vi "niDTS WLAN INSTR TX Configure ModAcc.vi"(8 "error in (no error)":errorcluster, 11 "niDTS WLAN INSTR TX in":refnum<class "niDTS WLAN INSTR TX.lvclass">) -> (0 "error out":errorcluster, 3 "niDTS WLAN INSTR TX out":refnum<class "niDTS WLAN INSTR TX.lvclass">)   [LabVIEW 2015, in "niDTS WLAN.lvlib" / "niDTS WLAN INSTR TX.lvclass"]
doc: "Sets:\n\n* ModulationEnabled\n* HeaderDetectionEnabled\n* AmplitudeTracking\n* ChannelTracking\n* TimeTracking\n* NumberOfAverages(mod)\n* PayloadLength\n\nNotes: This section is missing Number of Symbols to Analyze and L-SIG length."
uses:
  niDTS WLAN INSTR TX.lvclass
  niDTS WLAN INSTR TX.lvclass/niDTS WLAN INSTR TX.ctl
  RiviInstDriver/niRfsaWlan/Objects/niRfsaWlan.lvclass
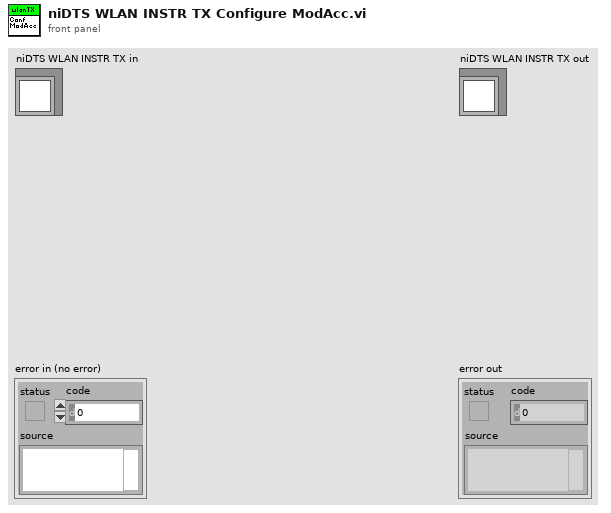
[diagram p1: front panel]
types:
  T1 = typedef "niDTS WLAN.lvlib/niDTS WLAN INC Standard.ctl" = enum16{"802.11 b DSSS", "802.11 a/g OFDM", "802.11 n HT", "802.11 ac VHT"}
  T2 = typedef "niRfsaWlan.lvclass/niRfsaWlan INC Handle.ctl" = refnum<data-value>
  T3 = typedef "niDTS WLAN.lvlib/niDTS WLAN INC DSSS ModAcc Measurement Parameters.ctl" = cluster{"DC Offset Compensation":bool, "Equalization":bool, "Phase Tracking":bool, "Chip Start Location":i16, "Max Chips Used":i16, "Pulse Shaping FilterType":T4, "Pulse Shaping Filter Coefficient":dbl}
  T4 = typedef "niDTS WLAN.lvlib/niDTS WLAN INC Pulse Shaping Filter Type.ctl" = enum16{"NONE", "RCOSINE", "RRCOSINE", "GAUSSIAN"}
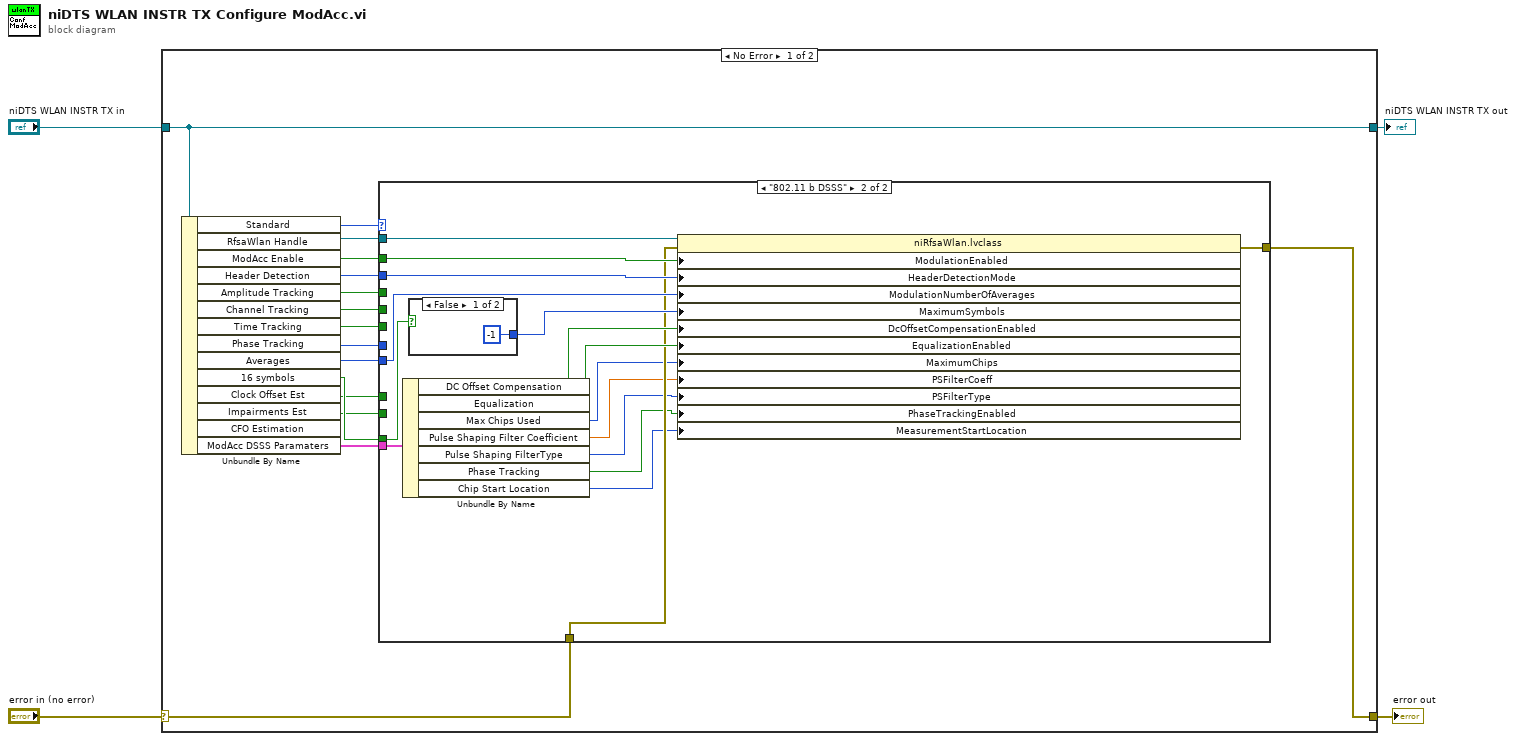
[diagram p0: block diagram]
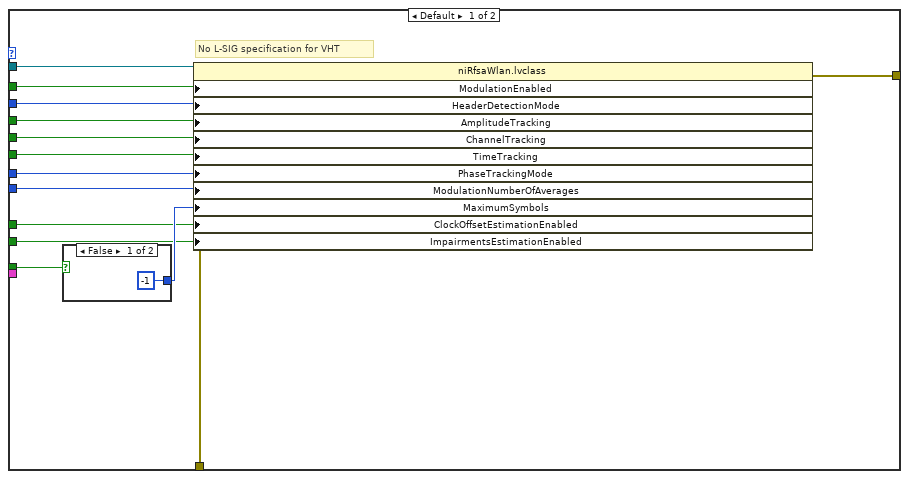
[diagram p2: hidden frame]
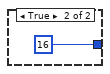
[diagram p3: hidden frame]
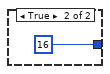
[diagram p4: hidden frame]
diagram:
  n1 = case shown="No Error" "error in (no error)" {
    selector: "error in (no error)" -> [w18 w56]
    tunnel: [w17 w56] -> w3
    tunnel: [w20 w55] -> w1
    tunnel: "niDTS WLAN INSTR TX in" -> [w20 w55]
    frame No Error {
      n2 = Unbundle By Name(w20) -> ("Standard"=w6:T1, "RfsaWlan Handle"=w19:T2, "ModAcc Enable"=w16:bool, "Header Detection"=w10:enum16{"MANUAL", "FIRST", "ALL"}, "Amplitude Tracking"=w15:bool, "Channel Tracking"=w14:bool, "Time Tracking"=w13:bool, "Phase Tracking"=w7:enum16{"NONE", "STANDARD", "CSF", "INSTANT"}, "Averages"=w12:i32, "16 symbols"=w11:bool, "Clock Offset Est"=w9:bool, "Impairments Est"=w8:bool, "ModAcc DSSS Paramaters"=w5:T3)  [unwired: 1 out]
      n3 = case shown="\"802.11 b DSSS\"" w6 {
        tunnel: w19 -> [w34 w52]
        tunnel: w18 -> [w33 w42]
        tunnel: [w32 w51] -> w17
        tunnel: w16 -> [w31 w50]
        tunnel: w15 -> [w30 _]
        tunnel: w14 -> [w29 _]
        tunnel: w13 -> [w28 _]
        tunnel: w12 -> [w27 w49]
        tunnel: w11 -> [w26 w48]
        tunnel: w10 -> [w24 w46]
        tunnel: w9 -> [w23 _]
        tunnel: w8 -> [w22 _]
        tunnel: w7 -> [w21 _]
        tunnel: w5 -> [_ w45]
        frame Default {
          # "No L-SIG specification for VHT"
          n4 = case shown="False" w26 {
            tunnel: [-1 16] -> w25
            frame False {
            }
            frame True {
            }
          }
          n5 = property class="niRfsaWlan.lvclass"(reference=w34, error in=w33, "ModulationEnabled"=w31, "HeaderDetectionMode"=w24, "AmplitudeTracking"=w30, "ChannelTracking"=w29, "TimeTracking"=w28, "PhaseTrackingMode"=w21, "ModulationNumberOfAverages"=w27, "MaximumSymbols"=w25, "ClockOffsetEstimationEnabled"=w23, "ImpairmentsEstimationEnabled"=w22) -> (error out=w32:errorcluster)  [unwired: 1 out]
        }
        frame "802.11 b DSSS" {
          n6 = Unbundle By Name(w45) -> ("DC Offset Compensation"=w44:bool, "Equalization"=w43:bool, "Max Chips Used"=w41:i16, "Pulse Shaping Filter Coefficient"=w40:dbl, "Pulse Shaping FilterType"=w39:T4, "Phase Tracking"=w38:bool, "Chip Start Location"=w37:i16)
          n7 = case shown="False" w48 {
            tunnel: [-1 16] -> w47
            frame False {
            }
            frame True {
            }
          }
          n8 = property class="niRfsaWlan.lvclass"(reference=w52, error in=w42, "ModulationEnabled"=w50, "HeaderDetectionMode"=w46, "ModulationNumberOfAverages"=w49, "MaximumSymbols"=w47, "DcOffsetCompensationEnabled"=w44, "EqualizationEnabled"=w43, "MaximumChips"=w41, "PSFilterCoeff"=w40, "PSFilterType"=w39, "PhaseTrackingEnabled"=w38, "MeasurementStartLocation"=w37) -> (error out=w51:errorcluster)  [unwired: 1 out]
        }
      }
    }
    frame Error {
    }
  }
  "error out" <- w3
  "niDTS WLAN INSTR TX out" <- w1
